vi "Read_Template.vi"(8 "error in (no error)":errorcluster, 11 "Class in":refnum<class "dsfsdfsd.lvclass">) -> (0 "error out":errorcluster, 2 "Control out":cluster{"Numeric":dbl, "String":string}[](array[cluster]), 3 "Class out":refnum<class "dsfsdfsd.lvclass">)   [LabVIEW 2013]
uses:
  TestProject/Class1/dsfsdfsd.lvclass
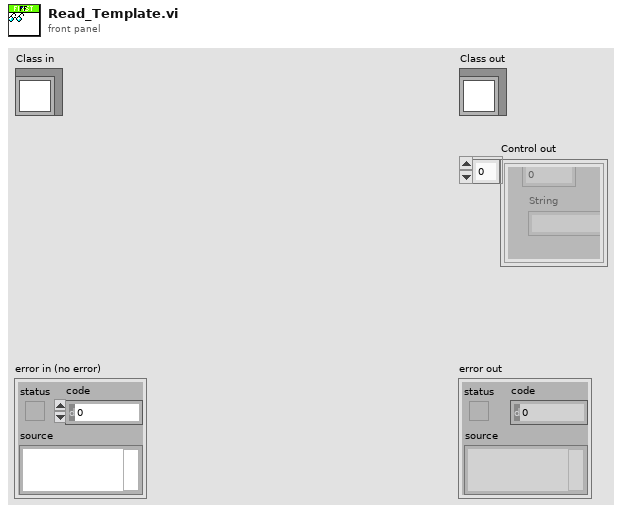
[diagram p1: front panel]
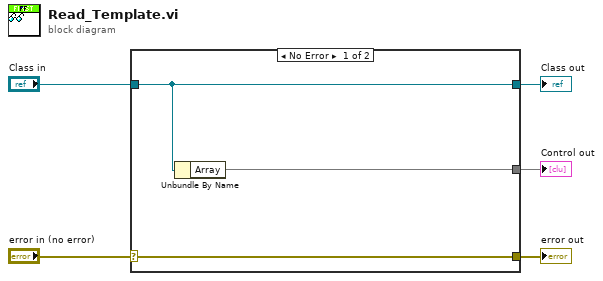
[diagram p0: block diagram]
diagram:
  n1 = case shown="No Error" "error in (no error)" {
    selector: "error in (no error)" -> [w8 w9]
    tunnel: [w8 w9] -> w4
    tunnel: [w7 w10] -> w2
    tunnel: "Class in" -> [w7 w10]
    tunnel: [w6 _] -> w1
    frame No Error {
      n2 = Unbundle By Name "Unbundle By Name"(w7) -> ("Array"=w6)
    }
    frame Error {
    }
  }
  "error out" <- w4
  "Class out" <- w2
  "Control out" <- w1
